vi "Main interface.vi"() -> ()   [LabVIEW 2017]
uses:
  <instrlib>/Harvard Apparatus PHD Ultra Series/Harvard Apparatus PHD Ultra Series.lvlib
  <instrlib>/Harvard Syringe Pump PHD2000/Harvard Syringe Pump PHD2000.lvlib
panel:
  in  "Main interface":T1(tab)
  in  "Acutally run actions":bool
  in  "Main interface stop":bool
  in  "Connection COM ports table":enum32{"Pump", "Potentiostat", "Rotation"}(tab)
  in  "Pump COM ports":T2={"Pump 1 COM"="COM11", "Pump 2 COM"="COM9", "Pump 3 COM"="", "Pump 4 COM"="COM4", "Pump 5 COM"="COM12"}
  in  "Enable potentiostat":bool
  in  "Potentiostat channel":string(combo)="17152001"
  in  "Enable rotation":bool
  in  "Rotation COM":refnum<visa-resource-name>="COM7"
  in  "Control parameters":T3(tab)
  in  "Purge control parameter":T4={"Pressure (psi)"=40.0, "Repeat times"=2, "Delayed time for waiting(s)"=5.0, "Refill rate\n(ml/min)"=3.0, "Refill volume (mL)"=2.5, "Infuse rate\n(ml/min)"=1.0, "Infuse volume (mL)"=2.5, "Sample loop prime volume (mL) "=0.6} {"Sample loop prime volume (mL)" format="%#.4f"; "Infuse volume (mL)" format="%#.4f"; "Infuse rate\n(ml/min)" format="%#.4f"; "Refill volume (mL)" format="%#.4f"; "Refill rate\n(ml/min)" format="%#.4f"}
  in  "Prime pumps":bool
  in  "Rinse control parameters":T5={"Pump 2 fill rate (ml/min)"=0.5, "Pump 2 rinse times"=1, "Pump 2 fill volume (ml)"=0.1, "Pump 1 rinse rate (ml/min)"=0.2, "Pump 1 rinse volume (mL)"=0.6, "Pump 1 fill volume (mL)"=0.6, "Pump 1 fill rate (ml/min)"=3.0, "Delayed time for waiting(s)"=5.0, "Pump 3 fill rate (ml/min)"=0.5, "Pump 3 fill volume (ml)"=0.1, "Pump 3 muliplier"=1.0, "Pump 3 rinse times"=1, "Gas purge muliplier"=1.5, "Gas purge?"=TRUE, "Pump 1 clear rate (ml/min)"=0.1, "Clear?"=FALSE, "Rinse injection order"=enum."Pump 2 first"} {"Pump 1 clear rate (ml/min)" format="%#.4f"; "Gas purge muliplier" min=0.0 max=50.0 format="%#.3g"; "Pump 3 muliplier" min=0.0 max=50.0 format="%#.3g"; "Pump 3 fill volume (ml)" min=0.0 max=50.0 format="%#.3g"; "Pump 3 fill rate (ml/min)" min=0.0 max=500.0 format="%#.3g"; "Pump 1 fill rate (ml/min)" format="%#.4f"; "Pump 1 fill volume (mL)" format="%#.4f"; "Pump 1 rinse volume (mL)" format="%#.4f"; "Pump 1 rinse rate (ml/min)" format="%#.4f"; "Pump 2 fill volume (ml)" min=0.0 max=50.0 format="%#.3g"; "Pump 2 fill rate (ml/min)" min=0.0 max=500.0 format="%#.3g"}
  in  "Syringe mode parameter":T6={"Pump 5 charge rate (ml/min)"=0.5, "Pump 5 charge volume (mL)"=0.1} {"Pump 5 charge volume (mL)" format="%#.4f"; "Pump 5 charge rate (ml/min)" format="%#.4f"}
  in  "ALS mode parameter":T7={"Wash vial Location"=106.0, "Reagent volume (ul)"=[25.0, 6.0, 19.0], "Reagent location"=[101.0, 103.0, 102.0], "Mix vial Location"=31.0, "Pump 5 target volume (ml)"=1.0, "Pump 5  flowrate (ml/min)"=0.15, "Sample name"="YM4-246-4"} {"Pump 5  flowrate (ml/min)" min=0.0 format="%#.4f"; "Pump 5 target volume (ml)" min=0.0 format="%#.4f"}
  in  "ChemStation Name":string="hpcore16444"
  in  "Connection type":enum16{"Local", "Remote"}(ring)
  in  "Reaction parameter":T8={"Pump 1 refill rate (ml/min) "=3.0, "Pump 1 refill volume (mL)"=0.8, "Pump 1 transfer rate (ml/min)"=0.12, "Pump 1 oscill. rate (ml/min)"=0.1, "Vertex potential 1(V)"=1.5, "Initial potential (V)"=0.0, "Final potential (V)"=0.0, "Cycles"=2, "Delayed time for waiting(s)"=5.0, "Pressure (psi)"=40.0, "Vertex potential 2(V)"=-0.1, "Use inital potential?"=TRUE, "Sample name"="YM4-246-4", "To waste flow factor"=3.0, "Temperature (C)"=20.0, "Scan rate (V/s)"=0.15, "Use final potential?"=TRUE, "CV current range"="2MA", "Cell to use"="EXTERNAL"} {"Scan rate (V/s)" min=0.0 max=10.0 format="%#_4f"; "Vertex potential 2(V)" min=-5.0 max=5.0 format="%.3f"; "Cycles" min=1 max=30; "Final potential (V)" min=-5.0 format="%_3f"; "Initial potential (V)" min=-5.0 max=5.0 format="%.3f"; "Vertex potential 1(V)" min=-5.0 max=5.0 format="%.3f"; "Pump 1 oscill. rate (ml/min)" format="%#.4f"; "Pump 1 transfer rate (ml/min)" format="%#.4f"; "Pump 1 refill volume (mL)" format="%#.4f"; "Pump 1 refill rate (ml/min)" format="%#.4f"}
  out "Valve 5":bool
  out "Voltage (V)":dbl
  out "Current (mA)":dbl
  out "Potentiostat set":bool
  out "Potentiostat start":bool
  out "Potentiostat running":bool
  out "DDE control":i8
  in  "Purge glove box":bool
  out "Sample name":string
  out "Pressure (psi)":dbl
  out "Temperature (C)":dbl
  out "Low voltage (V)":dbl
  out "High voltage (V)":dbl
  out "Scan rate (V//s)":dbl
  out "Reagent volume (ul)":dbl[](array[numeric])
  out "Connected":bool
  in  "Sample source":enum16{"Syringe", "ALS"}(ring)=enum."ALS"
  out "Action running":T9(ring)
  out "Time passed (min)":dbl
  out "Valve 4":bool
  out "Pressure gauage 2(psi)":dbl
  out "Pressure gauage 1(psi)":dbl
  out "Pump 1 position (ml)":dbl
  in  "Vaccum done?":bool
  out "Manual vaccum":bool
  in  "Emergence stop":bool
  in  "Action to run":T9(ring)
  in  "Start Exp.":bool
  in  "Experiments":bool
  out "Process running":bool
  out "Pressure value (psi)":dbl
  out "Pressure control (psi)":dbl
  out "ALS Ready":bool
  out "ALS START":bool
  out "HPLC START":bool
  out "HPLC Reday":bool
  out "Valve 3":bool
  out "Valve 2":bool
  out "Valve 1":bool
  out "Phase sensor digital":bool[](array[boolean])
  out "HPLC pressure (bar)":dbl
  in  "Exp. file path":path=path "C:/Users/Optix/Dropbox (MIT)/Research/Backup/66-225 Optix data/Yiming MO/Echem screening/Test experiment folder"
  in  "Experiment finished?":bool
  out "Sample index":i32
  in  "Experiment name":string="YM3-xxx"
  out "System status":string
  out "Reagent location":dbl[](array[numeric])
  out "Real time CV":cluster{dbl[], dbl[]}(graph)
  out "Final CV plot":cluster{dbl[], dbl[]}(graph)
  in  "Revolution (0-0.5)":dbl=0.25 min=0.0 max=0.5 format="%#.2g"
  in  "Direction":enum16{"Counter clock", "Clock"}(ring)
  in  "Manual control":bool
  out "Manual control status":string
  in  "Manual control parameter":T10={"Pump 1 control"={"Pump Direction"=0, "Flow rate (ml/min)"=1.0, "Target volum (ml)"=1.0, "Run"=FALSE}, "Pump 4 control"={"Pump Direction"=0, "Flow rate (ml/min)"=1.0, "Target volum (ml)"=1.0, "Run"=FALSE}, "Pump 2 control"={"Flowrate (ml/min)"=0.0, "Target volume (ml)"=0.0, "Run"=FALSE}, "Pump 5 control"={"Pump Direction"=0, "Flow rate (ml/min)"=1.0, "Target volum (ml)"=1.0, "Run"=FALSE}, "Pump 3 control"={"Flowrate (ml/min)"=0.0, "Target volume (ml)"=0.0, "Run"=FALSE}} {"Pump 3 control"."Target volume (ml)" min=0.0 max=50.0 format="%#.3g"; "Pump 3 control"."Flowrate (ml/min)" min=0.0 max=500.0 format="%#.3g"; "Pump 5 control"."Target volum (ml)" format="%#.4f"; "Pump 5 control"."Flow rate (ml/min)" format="%#.4f"; "Pump 5 control"."Pump Direction" items=["Infuse", "Withdraw"]; "Pump 2 control"."Target volume (ml)" min=0.0 max=50.0 format="%#.3g"; "Pump 2 control"."Flowrate (ml/min)" min=0.0 max=500.0 format="%#.3g"; "Pump 4 control"."Target volum (ml)" format="%#.4f"; "Pump 4 control"."Flow rate (ml/min)" format="%#.4f"; "Pump 4 control"."Pump Direction" items=["Infuse", "Withdraw"]; "Pump 1 control"."Target volum (ml)" format="%#.4f"; "Pump 1 control"."Flow rate (ml/min)" format="%#.4f"; "Pump 1 control"."Pump Direction" items=["Infuse", "Withdraw"]}
  in  "Rotate":bool
  in  "Rotation speed (RPM)":dbl=2.0 min=0.0 max=50.0 step=0.1 format="%#.2g"
  out "Experiment log":string
  out "Action log":string
  in  "Record action log":bool
  in  "ALS method folder":path=path "C:/Chem32 (new)/2/Methods/DropletSys.M"
  # "Designed by Yiming Mo\nv. 0.8\n10/2019"
  # "ChemStation control mode"
  # "Following is only for local:"
  # "type \"print _DDENAME$\" in ChemStation"
  # "Experiments control"
  # "System status"
  # "Manual control"
  # "Current experiment key parameters"
  # "Potentiostat status"
  # "Rotation platform"
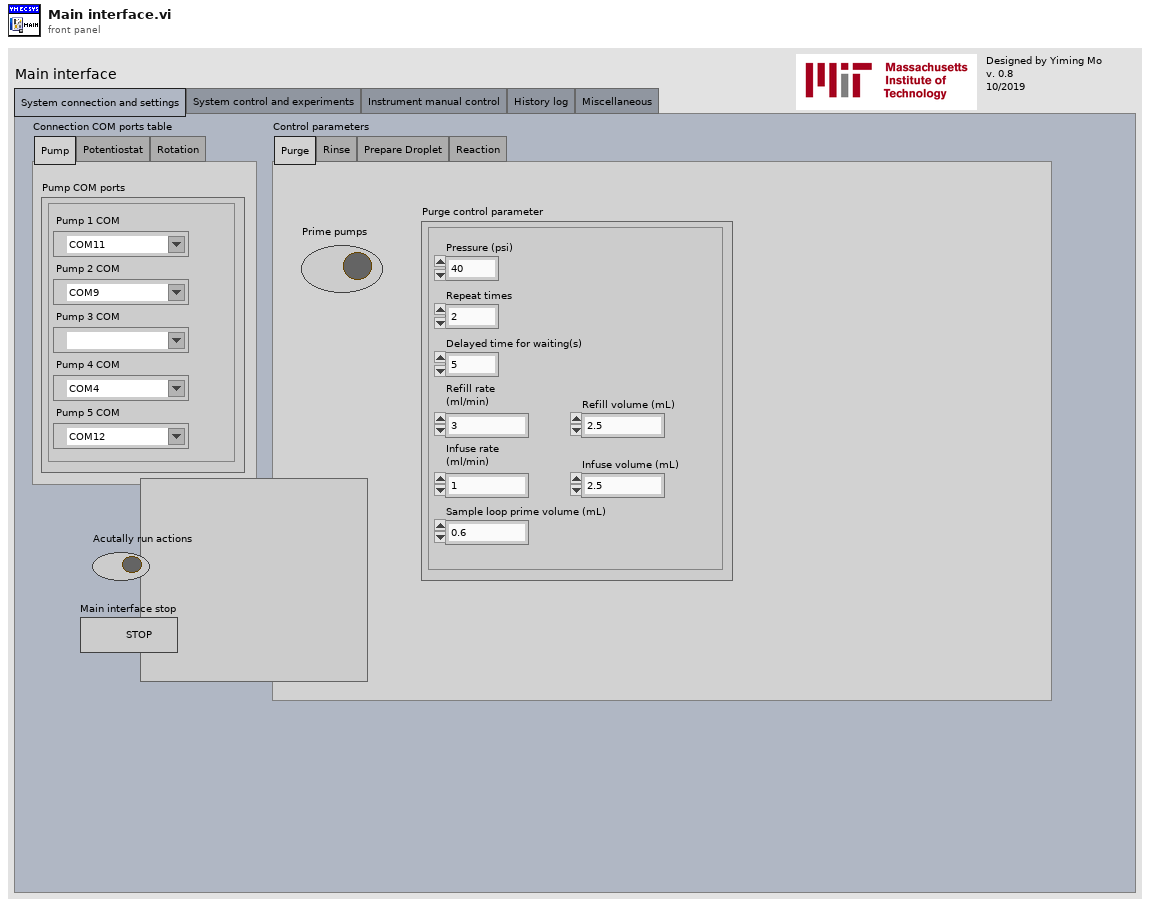
[diagram p1: front panel]
types:
  T1 = enum32{"System connection and settings", "System control and experiments", "Instrument manual control", "History log", "Miscellaneous"}
  T2 = cluster{"Pump 1 COM":refnum<visa-resource-name>, "Pump 2 COM":refnum<visa-resource-name>, "Pump 3 COM":refnum<visa-resource-name>, "Pump 4 COM":refnum<visa-resource-name>, "Pump 5 COM":refnum<visa-resource-name>}
  T3 = enum32{"Purge", "Rinse", "Prepare Droplet", "Reaction"}
  T4 = cluster{"Pressure (psi)":dbl, "Repeat times":i32, "Delayed time for waiting(s)":dbl, "Refill rate\n(ml/min)":dbl, "Refill volume (mL)":dbl, "Infuse rate\n(ml/min)":dbl, "Infuse volume (mL)":dbl, "Sample loop prime volume (mL) ":dbl}
  T5 = cluster{"Pump 2 fill rate (ml/min)":dbl, "Pump 2 rinse times":i32, "Pump 2 fill volume (ml)":dbl, "Pump 1 rinse rate (ml/min)":dbl, "Pump 1 rinse volume (mL)":dbl, "Pump 1 fill volume (mL)":dbl, "Pump 1 fill rate (ml/min)":dbl, "Delayed time for waiting(s)":dbl, "Pump 3 fill rate (ml/min)":dbl, "Pump 3 fill volume (ml)":dbl, "Pump 3 muliplier":dbl, "Pump 3 rinse times":i32, "Gas purge muliplier":dbl, "Gas purge?":bool, "Pump 1 clear rate (ml/min)":dbl, "Clear?":bool, "Rinse injection order":enum16{"Pump 2 first", "Pump 3 first"}}
  T6 = cluster{"Pump 5 charge rate (ml/min)":dbl, "Pump 5 charge volume (mL)":dbl}
  T7 = cluster{"Wash vial Location":dbl, "Reagent volume (ul)":dbl[], "Reagent location":dbl[], "Mix vial Location":dbl, "Pump 5 target volume (ml)":dbl, "Pump 5  flowrate (ml/min)":dbl, "Sample name":string}
  T8 = cluster{"Pump 1 refill rate (ml/min) ":dbl, "Pump 1 refill volume (mL)":dbl, "Pump 1 transfer rate (ml/min)":dbl, "Pump 1 oscill. rate (ml/min)":dbl, "Vertex potential 1(V)":dbl, "Initial potential (V)":dbl, "Final potential (V)":dbl, "Cycles":i32, "Delayed time for waiting(s)":dbl, "Pressure (psi)":dbl, "Vertex potential 2(V)":dbl, "Use inital potential?":bool, "Sample name":string, "To waste flow factor":dbl, "Temperature (C)":dbl, "Scan rate (V/s)":dbl, "Use final potential?":bool, "CV current range":string, "Cell to use":string}
  T9 = enum16{"0. Standby", "1. Purge with Argon", "2. Rinse with solvent", "3. Prepare droplet", "4. Reaction"}
  T10 = cluster{"Pump 1 control":cluster{"Pump Direction":u16, "Flow rate (ml/min)":dbl, "Target volum (ml)":dbl, "Run":bool}, "Pump 4 control":cluster{"Pump Direction":u16, "Flow rate (ml/min)":dbl, "Target volum (ml)":dbl, "Run":bool}, "Pump 2 control":cluster{"Flowrate (ml/min)":dbl, "Target volume (ml)":dbl, "Run":bool}, "Pump 5 control":cluster{"Pump Direction":u16, "Flow rate (ml/min)":dbl, "Target volum (ml)":dbl, "Run":bool}, "Pump 3 control":cluster{"Flowrate (ml/min)":dbl, "Target volume (ml)":dbl, "Run":bool}}
  T11 = enum32{"Invalid", "Standard", "Closed", "Hidden", "Minimized", "Maximized"}
  T12 = cluster{"Array of Double":dbl[], "Array of Double":dbl[]}
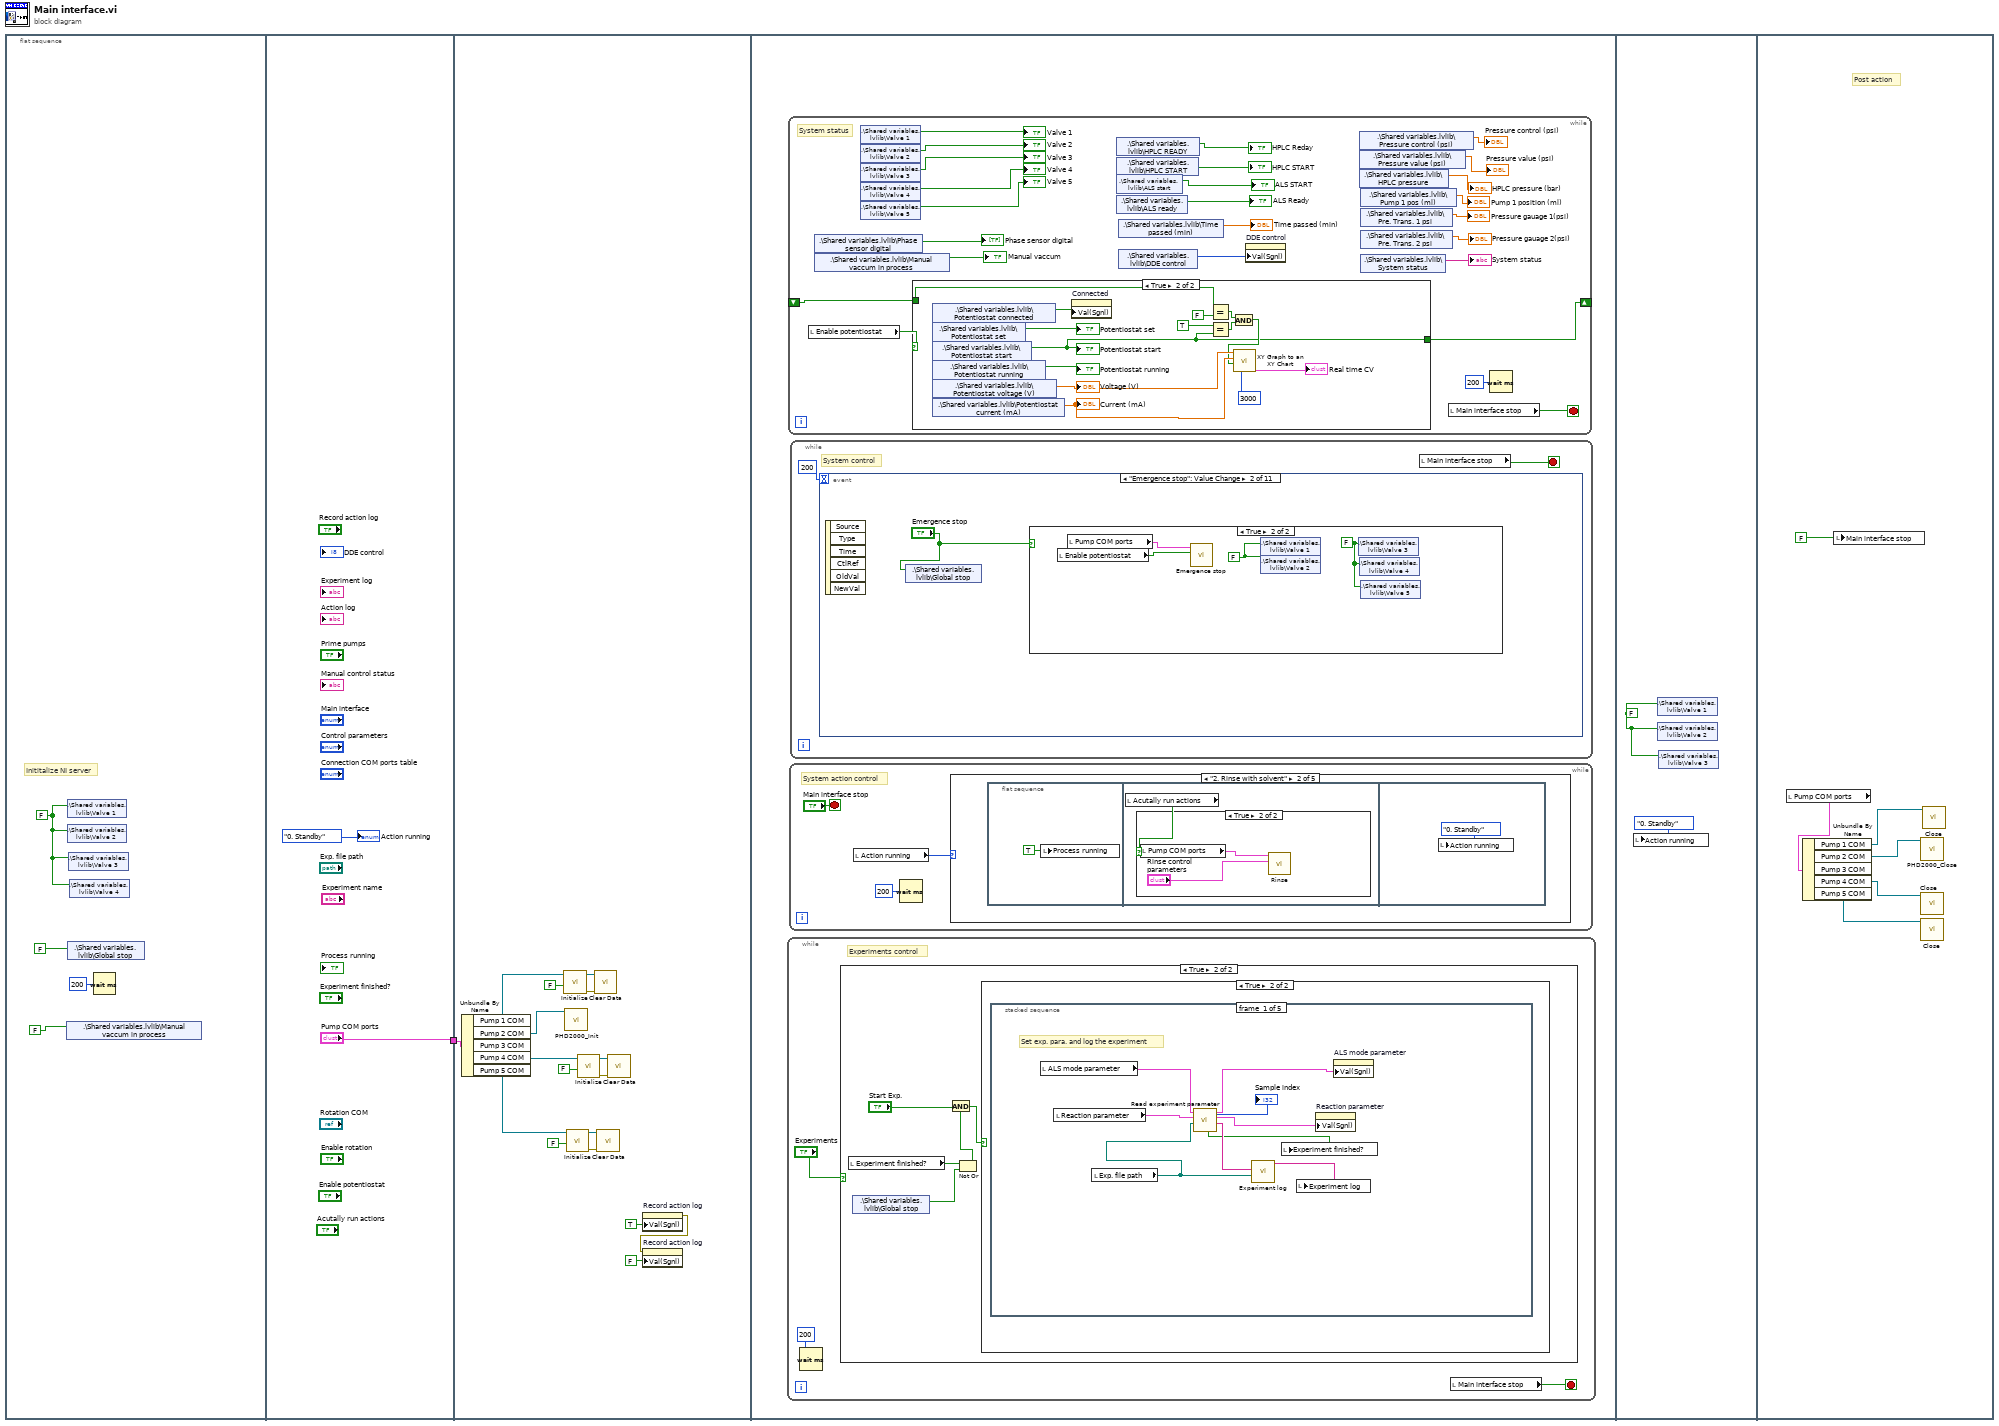
[diagram p0: block diagram]
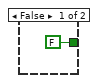
[diagram p2: hidden frame]
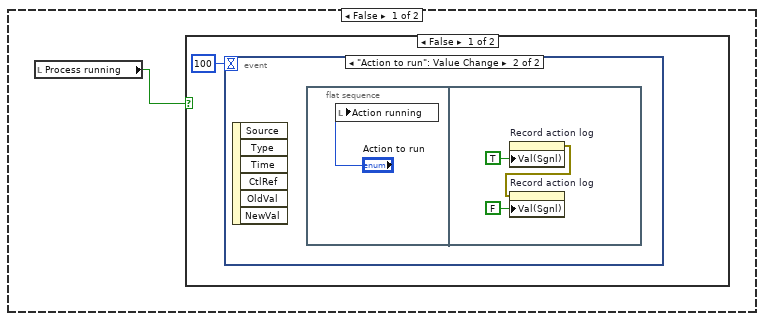
[diagram p3: hidden frame]
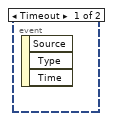
[diagram p4: hidden frame]
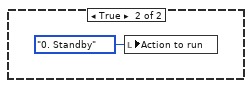
[diagram p5: hidden frame]
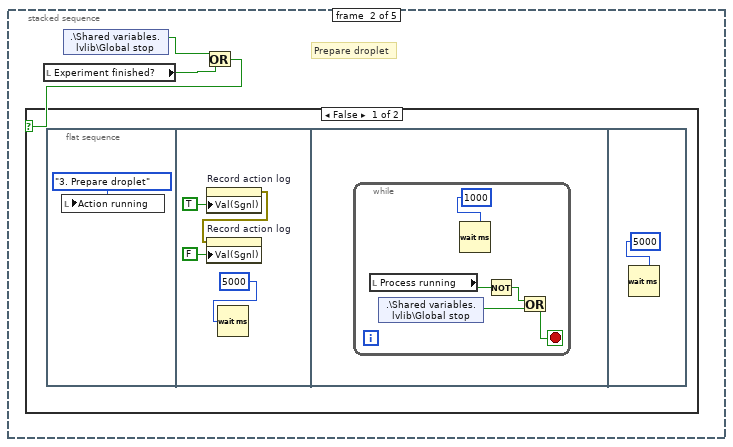
[diagram p7: hidden frame]
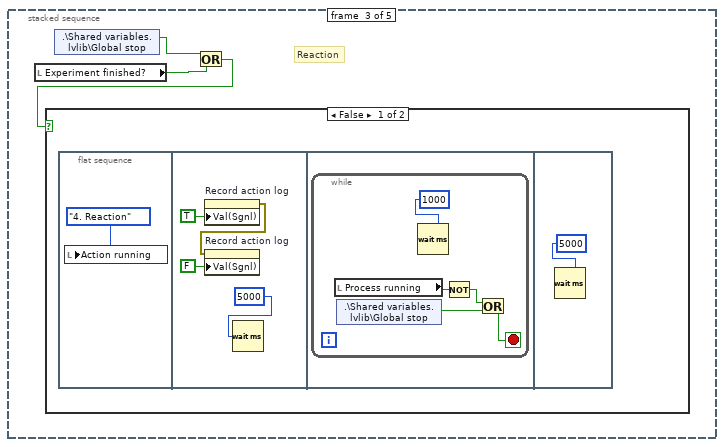
[diagram p9: hidden frame]
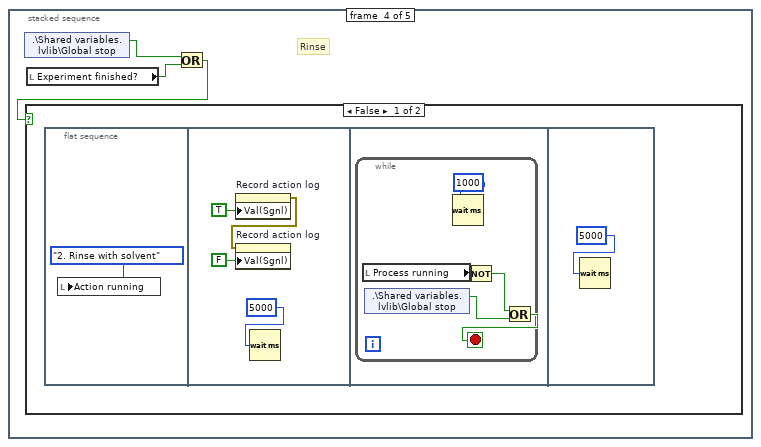
[diagram p11: hidden frame]
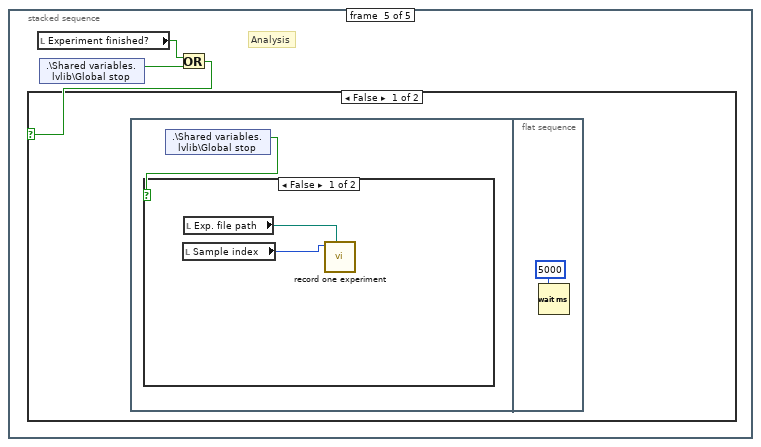
[diagram p13: hidden frame]
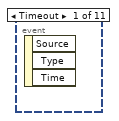
[diagram p16: hidden frame]
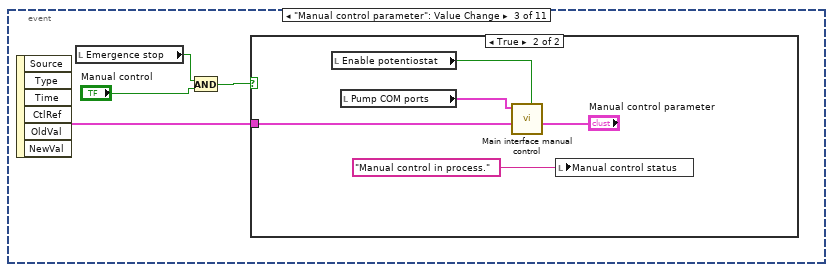
[diagram p18: hidden frame]
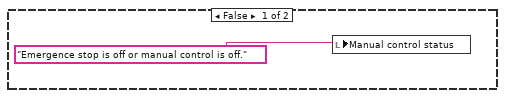
[diagram p19: hidden frame]
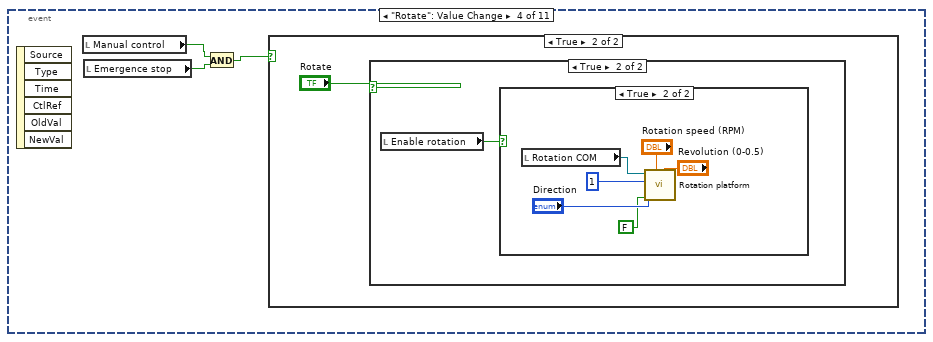
[diagram p20: hidden frame]
diagram:
  n1 = flat-sequence {
    tunnel: ["Pump COM ports"] -> w1
    tunnel: w1 -> [w24]
    frame #0 {
      w2 = FALSE
      # "Inititalize NI server"
      n2 = shared-variable ".\\Shared variables.lvlib\\Manual vaccum in process"(FALSE) -> ()  [unwired: 1 in, 1 out]
      n3 = shared-variable ".\\Shared variables.lvlib\\Valve 1"(w2) -> ()  [unwired: 1 in, 1 out]
      n4 = shared-variable ".\\Shared variables.lvlib\\Valve 2"(w2) -> ()  [unwired: 1 in, 1 out]
      n5 = shared-variable ".\\Shared variables.lvlib\\Global stop"(FALSE) -> ()  [unwired: 1 in, 1 out]
      n6 = shared-variable ".\\Shared variables.lvlib\\Valve 3"(w2) -> ()  [unwired: 1 in, 1 out]
      n7 = shared-variable ".\\Shared variables.lvlib\\Valve 4"(w2) -> ()  [unwired: 1 in, 1 out]
      n8 = Wait (ms)(milliseconds to wait=u32 200) -> ()  [unwired: 1 out]
    }
    frame #1 {
      "Action running" <- T9."0. Standby" ("Action running")
    }
    frame #2 {
      n9 = Unbundle By Name(w24) -> ("Pump 1 COM"=w21:refnum<visa-resource-name>, "Pump 2 COM"=w22:refnum<visa-resource-name>, "Pump 4 COM"=w23:refnum<visa-resource-name>, "Pump 5 COM"=w12:refnum<visa-resource-name>)  [unwired: 1 out]
      n10 = call <instrlib>:"Initialize.vi"("ID Query (True)"=FALSE, "VISA resource name"=w21) -> ("error out"=w18:errorcluster, "VISA resource name out"=w17:refnum<visa-resource-name>)  [unwired: 8 in]
      n11 = call <instrlib>:"PHD2000_Init.vi"("VISA resource name"=w22) -> ()  [unwired: 8 in, 2 out]
      n12 = call <instrlib>:"Initialize.vi"("ID Query (True)"=FALSE, "VISA resource name"=w12) -> ("error out"=w13:errorcluster, "VISA resource name out"=w11:refnum<visa-resource-name>)  [unwired: 8 in]
      n13 = call <instrlib>:"Initialize.vi"("ID Query (True)"=FALSE, "VISA resource name"=w23) -> ("error out"=w20:errorcluster, "VISA resource name out"=w19:refnum<visa-resource-name>)  [unwired: 8 in]
      n14 = call <instrlib>:"Clear Data.vi"("error in (no error)"=w18, "VISA resource name"=w17) -> ()  [unwired: 8 in, 2 out]
      n15 = call <instrlib>:"Clear Data.vi"("error in (no error)"=w13, "VISA resource name"=w11) -> ()  [unwired: 8 in, 2 out]
      n16 = call <instrlib>:"Clear Data.vi"("error in (no error)"=w20, "VISA resource name"=w19) -> ()  [unwired: 8 in, 2 out]
      n17 = property on="Record action log" class="Bool (strict)"("Val(Sgnl)"=TRUE ("Value (Signaling)")) -> (error out=w8:errorcluster)  [unwired: 2 in, 1 out]
      n18 = property on="Record action log" class="Bool (strict)"(error in=w8, "Val(Sgnl)"=FALSE ("Value (Signaling)")) -> ()  [unwired: 1 in, 2 out]
    }
    frame #3 {
      n19 = while {
        stop <- w66 stop-if-true
        # "Experiments control"
        n20 = Wait (ms)(milliseconds to wait=u32 200) -> ()  [unwired: 1 out]
        n21 = case shown="True" "Experiments" {
          frame False {
            n22 = local read "Process running"() -> (w68:bool)
            n23 = case shown="False" w68 {
              frame False {
                n24 = event shown="[1] \"Action to run\": Value Change" {
                  selector: _ -> [_ _]
                  dyn-events: _ -> [_ _]
                  timeout: 100 -> [_ _]
                  event Timeout {
                    n25 = event-data() -> ()  [unwired: 1 in, 3 out]
                  }
                  event "Action to run": Value Change {
                    n26 = event-data() -> ()  [unwired: 1 in, 6 out]
                    n27 = flat-sequence {
                      frame #0 {
                        n28 = local write "Action running"("Action to run") -> ()
                      }
                      frame #1 {
                        n29 = property on="Record action log" class="Bool (strict)"("Val(Sgnl)"=TRUE ("Value (Signaling)")) -> (error out=w73:errorcluster)  [unwired: 2 in, 1 out]
                        n30 = property on="Record action log" class="Bool (strict)"(error in=w73, "Val(Sgnl)"=FALSE ("Value (Signaling)")) -> ()  [unwired: 1 in, 2 out]
                      }
                    }
                  }
                }
              }
              frame True {
                n31 = local write "Action to run"(T9."0. Standby" ("Action to run")) -> ()
              }
            }
          }
          frame True {
            n32 = local read "Experiment finished?"() -> (w77:bool)
            n33 = shared-variable ".\\Shared variables.lvlib\\Global stop"() -> (w76:bool)  [unwired: 1 in, 1 out]
            n34 = Not Or(1:w76, 2:w77) -> (0:w78:bool)
            n35 = And(x="Start Exp.", y=w78) -> (x .and. y?=w75:bool)
            n36 = case shown="True" w75 {
              frame False {
              }
              frame True {
                n37 = stacked-sequence {
                  frame #0 {
                    # "Set exp. para. and log the experiment"
                    n38 = local read "ALS mode parameter"() -> (w87:T7)
                    n39 = local read "Reaction parameter"() -> (w83:T8)
                    n40 = local read "Exp. file path"() -> (w81:path)
                    n41 = call "Read experiment parameter.vi"("Exp. file path"=w81, "Reaction parameter in"=w83, "ALS mode parameter in"=w87) -> ("expInfo"=w86:string, "Reaction parameter out"=w82:T8, "ALS mode parameter out"=w80:T7, "Finished?"=w85:bool, "Index"=→"Sample index":i32)  [unwired: 3 in, 1 out]
                    n42 = call "Experiment log.vi"("file path (use dialog)"=w81, "New experiment info (from Matlab)"=w86) -> ("Experiment log out"=w88:string)  [unwired: 8 in, 1 out]
                    n43 = local write "Experiment finished?"(w85) -> ()
                    n44 = local write "Experiment log"(w88) -> ()
                    n45 = property on="Reaction parameter" class="Clust (strict)"("Val(Sgnl)"=w82) -> ()  [unwired: 2 in, 2 out]
                    n46 = property on="ALS mode parameter" class="Clust (strict)"("Val(Sgnl)"=w80) -> ()  [unwired: 2 in, 2 out]
                  }
                  frame #1 {
                    # "Prepare droplet"
                    n47 = local read "Experiment finished?"() -> (w90:bool)
                    n48 = shared-variable ".\\Shared variables.lvlib\\Global stop"() -> (w91:bool)  [unwired: 1 in, 1 out]
                    n49 = Or(x=w91, y=w90) -> (x .or. y?=w89:bool)
                    n50 = case shown="False" w89 {
                      frame False {
                        n51 = flat-sequence {
                          frame #0 {
                            n52 = local write "Action running"(T9."3. Prepare droplet" ("Action running")) -> ()
                          }
                          frame #1 {
                            n53 = property on="Record action log" class="Bool (strict)"("Val(Sgnl)"=TRUE ("Value (Signaling)")) -> (error out=w95:errorcluster)  [unwired: 2 in, 1 out]
                            n54 = property on="Record action log" class="Bool (strict)"(error in=w95, "Val(Sgnl)"=FALSE ("Value (Signaling)")) -> ()  [unwired: 1 in, 2 out]
                            n55 = Wait (ms)(milliseconds to wait=u32 5000) -> ()  [unwired: 1 out]
                          }
                          frame #2 {
                            n56 = while {
                              stop <- w99 stop-if-true
                              n57 = local read "Process running"() -> (w101:bool)
                              n58 = shared-variable ".\\Shared variables.lvlib\\Global stop"() -> (w98:bool)  [unwired: 1 in, 1 out]
                              n59 = Wait (ms)(milliseconds to wait=u32 1000) -> ()  [unwired: 1 out]
                              n60 = Not(x=w101) -> (.not. x?=w100:bool)
                              n61 = Or(x=w100, y=w98) -> (x .or. y?=w99:bool)
                            }
                          }
                          frame #3 {
                            n62 = Wait (ms)(milliseconds to wait=u32 5000) -> ()  [unwired: 1 out]
                          }
                        }
                      }
                      frame True {
                      }
                    }
                  }
                  frame #2 {
                    # "Reaction"
                    n63 = local read "Experiment finished?"() -> (w104:bool)
                    n64 = shared-variable ".\\Shared variables.lvlib\\Global stop"() -> (w105:bool)  [unwired: 1 in, 1 out]
                    n65 = Or(x=w105, y=w104) -> (x .or. y?=w103:bool)
                    n66 = case shown="False" w103 {
                      frame False {
                        n67 = flat-sequence {
                          frame #0 {
                            n68 = local write "Action running"(T9."4. Reaction" ("Action running")) -> ()
                          }
                          frame #1 {
                            n69 = property on="Record action log" class="Bool (strict)"("Val(Sgnl)"=TRUE ("Value (Signaling)")) -> (error out=w109:errorcluster)  [unwired: 2 in, 1 out]
                            n70 = property on="Record action log" class="Bool (strict)"(error in=w109, "Val(Sgnl)"=FALSE ("Value (Signaling)")) -> ()  [unwired: 1 in, 2 out]
                            n71 = Wait (ms)(milliseconds to wait=u32 5000) -> ()  [unwired: 1 out]
                          }
                          frame #2 {
                            n72 = while {
                              stop <- w113 stop-if-true
                              n73 = local read "Process running"() -> (w115:bool)
                              n74 = shared-variable ".\\Shared variables.lvlib\\Global stop"() -> (w112:bool)  [unwired: 1 in, 1 out]
                              n75 = Wait (ms)(milliseconds to wait=u32 1000) -> ()  [unwired: 1 out]
                              n76 = Not(x=w115) -> (.not. x?=w114:bool)
                              n77 = Or(x=w114, y=w112) -> (x .or. y?=w113:bool)
                            }
                          }
                          frame #3 {
                            n78 = Wait (ms)(milliseconds to wait=u32 5000) -> ()  [unwired: 1 out]
                          }
                        }
                      }
                      frame True {
                      }
                    }
                  }
                  frame #3 {
                    # "Rinse"
                    n79 = shared-variable ".\\Shared variables.lvlib\\Global stop"() -> (w119:bool)  [unwired: 1 in, 1 out]
                    n80 = local read "Experiment finished?"() -> (w118:bool)
                    n81 = Or(x=w119, y=w118) -> (x .or. y?=w117:bool)
                    n82 = case shown="False" w117 {
                      frame False {
                        n83 = flat-sequence {
                          frame #0 {
                            n84 = local write "Action running"(T9."2. Rinse with solvent" ("Action running")) -> ()
                          }
                          frame #1 {
                            n85 = property on="Record action log" class="Bool (strict)"("Val(Sgnl)"=TRUE ("Value (Signaling)")) -> (error out=w123:errorcluster)  [unwired: 2 in, 1 out]
                            n86 = property on="Record action log" class="Bool (strict)"(error in=w123, "Val(Sgnl)"=FALSE ("Value (Signaling)")) -> ()  [unwired: 1 in, 2 out]
                            n87 = Wait (ms)(milliseconds to wait=u32 5000) -> ()  [unwired: 1 out]
                          }
                          frame #2 {
                            n88 = while {
                              stop <- w128 stop-if-true
                              n89 = local read "Process running"() -> (w129:bool)
                              n90 = shared-variable ".\\Shared variables.lvlib\\Global stop"() -> (w127:bool)  [unwired: 1 in, 1 out]
                              n91 = Wait (ms)(milliseconds to wait=u32 1000) -> ()  [unwired: 1 out]
                              n92 = Not(x=w129) -> (.not. x?=w125:bool)
                              n93 = Or(x=w125, y=w127) -> (x .or. y?=w128:bool)
                            }
                          }
                          frame #3 {
                            n94 = Wait (ms)(milliseconds to wait=u32 5000) -> ()  [unwired: 1 out]
                          }
                        }
                      }
                      frame True {
                      }
                    }
                  }
                  frame #4 {
                    # "Analysis"
                    n95 = local read "Experiment finished?"() -> (w133:bool)
                    n96 = shared-variable ".\\Shared variables.lvlib\\Global stop"() -> (w132:bool)  [unwired: 1 in, 1 out]
                    n97 = Or(x=w133, y=w132) -> (x .or. y?=w131:bool)
                    n98 = case shown="False" w131 {
                      frame False {
                        n99 = flat-sequence {
                          frame #0 {
                            n100 = shared-variable ".\\Shared variables.lvlib\\Global stop"() -> (w134:bool)  [unwired: 1 in, 1 out]
                            n101 = case shown="False" w134 {
                              frame False {
                                n102 = local read "Sample index"() -> (w136:i32)
                                n103 = local read "Exp. file path"() -> (w135:path)
                                n104 = call "record one experiment.vi"("Exp. file path"=w135, "Sample index"=w136) -> ()  [unwired: 9 in, 1 out]
                              }
                              frame True {
                              }
                            }
                          }
                          frame #1 {
                            n105 = Wait (ms)(milliseconds to wait=u32 5000) -> ()  [unwired: 1 out]
                          }
                        }
                      }
                      frame True {
                      }
                    }
                  }
                }
              }
            }
          }
        }
        n106 = local read "Main interface stop"() -> (w66:bool)
      }
      n107 = while {
        shift-right: [w27] -> _
        shift-left: _ -> [w26]
        stop <- w49 stop-if-true
        # "System status"
        n108 = local read "Enable potentiostat"() -> (w28:bool)
        n109 = shared-variable ".\\Shared variables.lvlib\\Phase sensor digital"() -> (→"Phase sensor digital":bool[])  [unwired: 1 in, 1 out]
        n110 = shared-variable ".\\Shared variables.lvlib\\Manual vaccum in process"() -> (→"Manual vaccum":bool)  [unwired: 1 in, 1 out]
        n111 = shared-variable ".\\Shared variables.lvlib\\Valve 1"() -> (→"Valve 1":bool)  [unwired: 1 in, 1 out]
        n112 = shared-variable ".\\Shared variables.lvlib\\Valve 2"() -> (→"Valve 2":bool)  [unwired: 1 in, 1 out]
        n113 = shared-variable ".\\Shared variables.lvlib\\Valve 3"() -> (→"Valve 3":bool)  [unwired: 1 in, 1 out]
        n114 = shared-variable ".\\Shared variables.lvlib\\Valve 4"() -> (→"Valve 4":bool)  [unwired: 1 in, 1 out]
        n115 = shared-variable ".\\Shared variables.lvlib\\Valve 5"() -> (→"Valve 5":bool)  [unwired: 1 in, 1 out]
        n116 = case shown="True" w28 {
          tunnel: [FALSE ("Boolean") w56] -> w27
          tunnel: w26 -> [_ w57]
          frame False {
          }
          frame True {
            n117 = shared-variable ".\\Shared variables.lvlib\\Potentiostat connected"() -> (w52:bool)  [unwired: 1 in, 1 out]
            n118 = shared-variable ".\\Shared variables.lvlib\\Potentiostat set"() -> (→"Potentiostat set":bool)  [unwired: 1 in, 1 out]
            n119 = shared-variable ".\\Shared variables.lvlib\\Potentiostat start"() -> (w56:bool)  [unwired: 1 in, 1 out]
            "Potentiostat start" <- w56
            n120 = shared-variable ".\\Shared variables.lvlib\\Potentiostat running"() -> (→"Potentiostat running":bool)  [unwired: 1 in, 1 out]
            n121 = shared-variable ".\\Shared variables.lvlib\\Potentiostat voltage (V)"() -> (w62:dbl)  [unwired: 1 in, 1 out]
            "Voltage (V)" <- w62
            n122 = shared-variable ".\\Shared variables.lvlib\\Potentiostat current (mA)"() -> (w61:dbl)  [unwired: 1 in, 1 out]
            "Current (mA)" <- w61
            n123 = property on="Connected" class="Bool (strict)"("Val(Sgnl)"=w52) -> ()  [unwired: 2 in, 2 out]
            n124 = Equal?(x=w57, y=FALSE) -> (x = y?=w60:bool)
            n125 = Equal?(x=TRUE, y=w56) -> (x = y?=w59:bool)
            n126 = And(x=w60, y=w59) -> (x .and. y?=w58:bool)
            n127 = call "XY Graph to an XY Chart.vi"("Chart History (10,000)"=3000, "Clear Graph?"=w58, "Y Value"=w61, "X Value"=w62) -> ("XY Graph"=→"Real time CV":cluster{dbl[], dbl[]})  [unwired: 7 in]
          }
        }
        n128 = shared-variable ".\\Shared variables.lvlib\\HPLC READY"() -> (→"HPLC Reday":bool)  [unwired: 1 in, 1 out]
        n129 = shared-variable ".\\Shared variables.lvlib\\HPLC START"() -> (→"HPLC START":bool)  [unwired: 1 in, 1 out]
        n130 = shared-variable ".\\Shared variables.lvlib\\ALS start"() -> (→"ALS START":bool)  [unwired: 1 in, 1 out]
        n131 = shared-variable ".\\Shared variables.lvlib\\ALS ready"() -> (→"ALS Ready":bool)  [unwired: 1 in, 1 out]
        n132 = shared-variable ".\\Shared variables.lvlib\\Time passed (min)"() -> (→"Time passed (min)":dbl)  [unwired: 1 in, 1 out]
        n133 = shared-variable ".\\Shared variables.lvlib\\DDE control"() -> (w29:i8)  [unwired: 1 in, 1 out]
        n134 = property on="DDE control" class="DigNum (strict)"("Val(Sgnl)"=w29) -> ()  [unwired: 2 in, 2 out]
        n135 = shared-variable ".\\Shared variables.lvlib\\Pressure control (psi)"() -> (→"Pressure control (psi)":dbl)  [unwired: 1 in, 1 out]
        n136 = shared-variable ".\\Shared variables.lvlib\\Pressure value (psi)"() -> (→"Pressure value (psi)":dbl)  [unwired: 1 in, 1 out]
        n137 = shared-variable ".\\Shared variables.lvlib\\HPLC pressure"() -> (→"HPLC pressure (bar)":dbl)  [unwired: 1 in, 1 out]
        n138 = shared-variable ".\\Shared variables.lvlib\\Pump 1 pos (ml)"() -> (→"Pump 1 position (ml)":dbl)  [unwired: 1 in, 1 out]
        n139 = shared-variable ".\\Shared variables.lvlib\\Pre. Trans. 1 psi"() -> (→"Pressure gauage 1(psi)":dbl)  [unwired: 1 in, 1 out]
        n140 = shared-variable ".\\Shared variables.lvlib\\Pre. Trans. 2 psi"() -> (→"Pressure gauage 2(psi)":dbl)  [unwired: 1 in, 1 out]
        n141 = shared-variable ".\\Shared variables.lvlib\\System status"() -> (→"System status":string)  [unwired: 1 in, 1 out]
        n142 = local read "Main interface stop"() -> (w49:bool)
        n143 = Wait (ms)(milliseconds to wait=u32 200) -> ()  [unwired: 1 out]
      }
      n144 = while {
        stop <- "Main interface stop" stop-if-true
        # "System action control"
        n145 = local read "Action running"() -> (w212:T9)
        n146 = Wait (ms)(milliseconds to wait=u32 200) -> ()  [unwired: 1 out]
        n147 = case shown="\"2. Rinse with solvent\"" w212 {
          frame "1. Purge with Argon" {
            n148 = flat-sequence {
              frame #0 {
                n149 = local write "Process running"(TRUE ("Process running")) -> ()
              }
              frame #1 {
                n150 = local read "Acutally run actions"() -> (w215:bool)
                n151 = case shown="False" w215 {
                  frame False {
                    n152 = shared-variable ".\\Shared variables.lvlib\\System status"("1. test purge with Argon" ("System status")) -> ()  [unwired: 1 in, 1 out]
                    n153 = Wait (ms)(milliseconds to wait=u32 3000) -> ()  [unwired: 1 out]
                  }
                  frame True {
                    n154 = local read "Pump COM ports"() -> (w218:T2)
                    n155 = local read "Prime pumps"() -> (w219:bool)
                    n156 = call "Purge with argon.vi"("Prime pumps"=w219, "Control parameter"="Purge control parameter", "Configured COM ports"=w218) -> ()  [unwired: 9 in]
                  }
                }
              }
              frame #2 {
                n157 = local write "Action running"(T9."0. Standby" ("Action running")) -> ()
              }
            }
          }
          frame "2. Rinse with solvent" {
            n158 = flat-sequence {
              frame #0 {
                n159 = local write "Process running"(TRUE ("Process running")) -> ()
              }
              frame #1 {
                n160 = local read "Acutally run actions"() -> (w223:bool)
                n161 = case shown="True" w223 {
                  frame False {
                    n162 = shared-variable ".\\Shared variables.lvlib\\System status"("2. rinse with solvent" ("System status")) -> ()  [unwired: 1 in, 1 out]
                    n163 = Wait (ms)(milliseconds to wait=u32 3000) -> ()  [unwired: 1 out]
                  }
                  frame True {
                    n164 = local read "Pump COM ports"() -> (w226:T2)
                    n165 = call "Rinse.vi"("Control parameters"="Rinse control parameters", "Configured COM ports"=w226) -> ()  [unwired: 10 in]
                  }
                }
              }
              frame #2 {
                n166 = local write "Action running"(T9."0. Standby" ("Action running")) -> ()
              }
            }
          }
          frame "3. Prepare droplet" {
            n167 = flat-sequence {
              frame #0 {
                n168 = local write "Process running"(TRUE ("Process running")) -> ()
              }
              frame #1 {
                n169 = local read "Acutally run actions"() -> (w230:bool)
                n170 = case shown="True" w230 {
                  frame False {
                    n171 = shared-variable ".\\Shared variables.lvlib\\System status"("3. test prepare droplet" ("System status")) -> ()  [unwired: 1 in, 1 out]
                    n172 = Wait (ms)(milliseconds to wait=u32 3000) -> ()  [unwired: 1 out]
                  }
                  frame True {
                    n173 = local read "Pump COM ports"() -> (w234:T2)
                    n174 = local read "Exp. file path"() -> (w238:path)
                    n175 = call "Sample preparation.vi"("ALS mode parameter"="ALS mode parameter", "Syringe mode parameter"="Syringe mode parameter", "Sample source"="Sample source", "Experiment file path"=w238, "Method folder"="ALS method folder", "Configured COM ports"=w234) -> ()  [unwired: 6 in]
                  }
                }
              }
              frame #2 {
                n176 = local write "Action running"(T9."0. Standby" ("Action running")) -> ()
              }
            }
          }
          frame "4. Reaction" {
            n177 = flat-sequence {
              frame #0 {
                n178 = local write "Process running"(TRUE ("Process running")) -> ()
              }
              frame #1 {
                n179 = local read "Acutally run actions"() -> (w241:bool)
                n180 = case shown="True" w241 {
                  frame False {
                    n181 = shared-variable ".\\Shared variables.lvlib\\System status"("4. test reaction" ("System status")) -> ()  [unwired: 1 in, 1 out]
                    n182 = Wait (ms)(milliseconds to wait=u32 3000) -> ()  [unwired: 1 out]
                  }
                  frame True {
                    n183 = local read "Enable rotation"() -> (w244:bool)
                    n184 = local read "Rotation COM"() -> (w245:refnum<visa-resource-name>)
                    n185 = local read "Exp. file path"() -> (w249:path)
                    n186 = local read "Enable potentiostat"() -> (w250:bool)
                    n187 = local read "Pump COM ports"() -> (w248:T2)
                    n188 = call "Reaction.vi"("Enable potentiostat"=w250, "Experiment file path"=w249, "Potentiostat channel"="Potentiostat channel", "Enable rotation"=w244, "Rotation COM"=w245, "Control parameter"="Reaction parameter", "Configured COM ports"=w248) -> ()  [unwired: 5 in]
                  }
                }
              }
              frame #2 {
                n189 = local write "Action running"(T9."0. Standby" ("Action running")) -> ()
              }
            }
          }
          frame "0. Standby", Default {
            n190 = local write "Process running"(FALSE ("Process running")) -> ()
            n191 = shared-variable ".\\Shared variables.lvlib\\System status"("0. Standby") -> ()  [unwired: 1 in, 1 out]
          }
        }
      }
      n192 = while {
        stop <- w139 stop-if-true
        # "System control"
        n193 = event shown="[1] \"Emergence stop\": Value Change" {
          selector: _ -> [_ _ _ _ _ _ _ _ _ _ _]
          dyn-events: _ -> [_ _ _ _ _ _ _ _ _ _ _]
          timeout: 200 -> [_ _ _ _ _ _ _ _ _ _ _]
          event Timeout {
            n194 = event-data() -> ()  [unwired: 1 in, 3 out]
          }
          event "Emergence stop": Value Change {
            n195 = event-data() -> ()  [unwired: 1 in, 6 out]
            n196 = shared-variable ".\\Shared variables.lvlib\\Global stop"("Emergence stop") -> ()  [unwired: 1 in, 1 out]
            n197 = case shown="True" "Emergence stop" {
              frame False {
              }
              frame True {
                w141 = FALSE ("Valve 3")
                w144 = FALSE
                n198 = local read "Enable potentiostat"() -> (w143:bool)
                n199 = local read "Pump COM ports"() -> (w142:T2)
                n200 = call "Emergence stop.vi"("Enable potentiostat"=w143, "Configured COM ports"=w142) -> ()  [unwired: 10 in]
                n201 = shared-variable ".\\Shared variables.lvlib\\Valve 1"(w144) -> ()  [unwired: 1 in, 1 out]
                n202 = shared-variable ".\\Shared variables.lvlib\\Valve 2"(w144) -> ()  [unwired: 1 in, 1 out]
                n203 = shared-variable ".\\Shared variables.lvlib\\Valve 3"(w141) -> ()  [unwired: 1 in, 1 out]
                n204 = shared-variable ".\\Shared variables.lvlib\\Valve 4"(w141) -> ()  [unwired: 1 in, 1 out]
                n205 = shared-variable ".\\Shared variables.lvlib\\Valve 5"(w141) -> ()  [unwired: 1 in, 1 out]
              }
            }
          }
          event "Manual control parameter": Value Change {
            n206 = event-data() -> ("OldVal"=w145:T10)  [unwired: 1 in, 5 out]
            n207 = local read "Emergence stop"() -> (w146:bool)
            n208 = And(x=w146, y="Manual control") -> (x .and. y?=w148:bool)
            n209 = case shown="True" w148 {
              tunnel: w145 -> [_ w150]
              frame False {
                n210 = local write "Manual control status"("Emergence stop is off or manual control is off." ("Status ring")) -> ()
              }
              frame True {
                n211 = local read "Enable potentiostat"() -> (w152:bool)
                n212 = local read "Pump COM ports"() -> (w153:T2)
                n213 = call "Main interface manual control.vi"("Current"="Manual control parameter", "Enable potentiostat"=w152, "Previous"=w150, "Configured COM ports"=w153) -> ()  [unwired: 8 in]
                n214 = local write "Manual control status"("Manual control in process." ("Manual control status")) -> ()
              }
            }
          }
          event "Rotate": Value Change {
            n215 = event-data() -> ()  [unwired: 1 in, 6 out]
            n216 = local read "Manual control"() -> (w157:bool)
            n217 = local read "Emergence stop"() -> (w156:bool)
            n218 = And(x=w157, y=w156) -> (x .and. y?=w155:bool)
            n219 = case shown="True" w155 {
              frame False {
              }
              frame True {
                n220 = case shown="True" "Rotate" {
                  frame False {
                  }
                  frame True {
                    n221 = local read "Enable rotation"() -> (w159:bool)
                    n222 = case shown="True" w159 {
                      frame False {
                      }
                      frame True {
                        n223 = local read "Rotation COM"() -> (w165:refnum<visa-resource-name>)
                        n224 = call "Rotation platform.vi"("Revolution (0-0.5)"="Revolution (0-0.5)", "Rotation speed (RPM)"="Rotation speed (RPM)", "Wait?"=FALSE, "Direction"="Direction", "Pump number"=1, "Rotation COM"=w165) -> ()  [unwired: 6 in]
                      }
                    }
                  }
                }
              }
            }
          }
          event "Vaccum done?": Value Change {
            n225 = event-data() -> ()  [unwired: 1 in, 6 out]
            n226 = case shown="True" "Vaccum done?" {
              frame False {
              }
              frame True {
                n227 = flat-sequence {
                  frame #0 {
                    n228 = shared-variable ".\\Shared variables.lvlib\\Maual vaccum done?"(TRUE) -> ()  [unwired: 1 in, 1 out]
                  }
                  frame #1 {
                    n229 = Wait (ms)(milliseconds to wait=u32 2000) -> ()  [unwired: 1 out]
                  }
                  frame #2 {
                    w169 = FALSE
                    n230 = shared-variable ".\\Shared variables.lvlib\\Maual vaccum done?"(w169) -> ()  [unwired: 1 in, 1 out]
                    n231 = local write "Vaccum done?"(w169) -> ()
                  }
                }
              }
            }
          }
          event "Record action log": Value Change {
            # "Action log"
            n232 = event-data() -> ("NewVal"=w170:bool)  [unwired: 1 in, 5 out]
            n233 = case shown="True" w170 {
              frame False {
              }
              frame True {
                n234 = local read "Action running"() -> (w173:T9)
                n235 = local read "Exp. file path"() -> (w171:path)
                n236 = call "Action log.vi"("file path (use dialog)"=w171, "Action running"=w173) -> ("Action log out"=w172:string)  [unwired: 8 in, 1 out]
                n237 = local write "Action log"(w172) -> ()
              }
            }
          }
          event "Reaction parameter": Value Change {
            # "Update current experiment (auto and manual) key parameters"
            n238 = event-data() -> ()  [unwired: 1 in, 6 out]
            n239 = local read "Reaction parameter"() -> (w180:T8)
            n240 = Unbundle By Name(w180) -> ("Sample name"=w174:string, "Pressure (psi)"=→"Pressure (psi)":dbl, "Temperature (C)"=→"Temperature (C)":dbl, "Vertex potential 1(V)"=→"Low voltage (V)":dbl, "Vertex potential 2(V)"=→"High voltage (V)":dbl, "Scan rate (V/s)"=→"Scan rate (V//s)":dbl)
            n241 = local read "ALS mode parameter"() -> (w182:T7)
            n242 = local write "Experiment name"(w174) -> ()
            n243 = Bundle By Name(cluster=w182, "Sample name"=w174) -> (w181:T7)
            n244 = local write "ALS mode parameter"(w181) -> ()
          }
          event "ALS mode parameter": Value Change {
            # "Update current experiment (auto and manual) key parameters"
            n245 = event-data() -> ()  [unwired: 1 in, 6 out]
            n246 = local read "ALS mode parameter"() -> (w186:T7)
            n247 = local read "Reaction parameter"() -> (w185:T8)
            n248 = Unbundle By Name(w186) -> ("Sample name"=w183:string, "Reagent location"=→"Reagent location":dbl[], "Reagent volume (ul)"=→"Reagent volume (ul)":dbl[])
            "Sample name" <- w183
            n249 = Bundle By Name(cluster=w185, "Sample name"=w183) -> (w184:T8)
            n250 = local write "Experiment name"(w183) -> ()
            n251 = local write "Reaction parameter"(w184) -> ()
          }
          event "Purge glove box": Value Change {
            n252 = event-data() -> ()  [unwired: 1 in, 6 out]
            n253 = case shown="True" "Purge glove box" {
              frame False {
              }
              frame True {
                n254 = Current VI's Path() -> (path=w199:path)
                n255 = Strip Path(path=w199) -> (stripped path=w198:path)  [unwired: 1 out]
                n256 = Build Path(base path=w198, name or relative path="Glove box startup.vi") -> (appended path=w196:path)
                n257 = Open VI Reference(vi path=w196) -> (vi reference=w195:refnum<vi>, error out=w191:errorcluster)  [unwired: 5 in]
                n258 = invoke class="VI" method="FP.Open"(reference=w195, error in=w191, "Activate"=TRUE ("Activate?"), "State"=T11."Standard") -> (reference out=w192:refnum<vi>, error out=w190:errorcluster)  [unwired: 1 in, 3 out]
                n259 = Close Reference(reference=w192, error in (no error)=w190) -> ()  [unwired: 1 out]
              }
            }
          }
          event "DDE control": Value Change {
            # "ChemStation\nDDE control"
            n260 = event-data() -> ()  [unwired: 1 in, 6 out]
            n261 = case shown="\"Local\", Default" "Connection type" {
              frame "Local", Default {
                n262 = shared-variable ".\\Shared variables.lvlib\\DDE control"() -> (w201:i8)  [unwired: 1 in, 1 out]
                n263 = Not Equal?(x=w201, y=i8 0) -> (x != y?=w203:bool)
                n264 = case shown="True" w203 {
                  tunnel: w201 -> [_ w204]
                  frame False {
                  }
                  frame True {
                    n265 = local read "ALS method folder"() -> (w206:path)
                    n266 = call "ALS control local.vi"("DDE control"=w204, "ChemStation Name"="ChemStation Name", "ALS method folder"=w206) -> ()  [unwired: 8 in]
                  }
                }
              }
              frame "Remote" {
              }
            }
          }
          event "Connected": Value Change {
            n267 = event-data() -> ("NewVal"=w207:bool)  [unwired: 1 in, 5 out]
            n268 = case shown="False" w207 {
              frame False {
                n269 = shared-variable ".\\Shared variables.lvlib\\CV voltage"() -> (w210:dbl[])  [unwired: 1 in, 1 out]
                n270 = shared-variable ".\\Shared variables.lvlib\\CV current"() -> (w209:dbl[])  [unwired: 1 in, 1 out]
                n271 = Bundle("Array of Double"=w210, "Array of Double"=w209) -> (→"Final CV plot":T12)  [unwired: 1 in]
              }
              frame True {
              }
            }
          }
        }
        n272 = local read "Main interface stop"() -> (w139:bool)
      }
    }
    frame #4 {
      w255 = FALSE
      n273 = local write "Action running"(T9."0. Standby" ("Action running")) -> ()
      n274 = shared-variable ".\\Shared variables.lvlib\\Valve 1"(w255) -> ()  [unwired: 1 in, 1 out]
      n275 = shared-variable ".\\Shared variables.lvlib\\Valve 2"(w255) -> ()  [unwired: 1 in, 1 out]
      n276 = shared-variable ".\\Shared variables.lvlib\\Valve 3"(w255) -> ()  [unwired: 1 in, 1 out]
    }
    frame #5 {
      # "Post action"
      n277 = local read "Pump COM ports"() -> (w260:T2)
      n278 = Unbundle By Name(w260) -> ("Pump 1 COM"=w259:refnum<visa-resource-name>, "Pump 2 COM"=w258:refnum<visa-resource-name>, "Pump 4 COM"=w257:refnum<visa-resource-name>, "Pump 5 COM"=w256:refnum<visa-resource-name>)  [unwired: 1 out]
      n279 = local write "Main interface stop"(FALSE) -> ()
      n280 = call <instrlib>:"PHD2000_Close.vi"("VISA resource name"=w258) -> ()  [unwired: 9 in, 1 out]
      n281 = call <instrlib>:"Close.vi"("VISA resource name"=w257) -> ()  [unwired: 10 in, 1 out]
      n282 = call <instrlib>:"Close.vi"("VISA resource name"=w256) -> ()  [unwired: 10 in, 1 out]
      n283 = call <instrlib>:"Close.vi"("VISA resource name"=w259) -> ()  [unwired: 10 in, 1 out]
    }
  }
